vi "franch_sliding_correlator.vi"(4 "error in (no error)":errorcluster, 5 "modulation parameters":T1={"modulation type"="QPSK", "pulse shaping parameters"={"modulation type"=enum."PSK", "pulse shaping filter"=enum."Root Raised Cos", "filter parameter"=0.5, "filter length (symbols)"=8}, "control information\nfor packet header/tail"={"Training Sequence (derived)"=[0.7071067811865475+0.7071067811865475i, 0.7071067811865475+0.7071067811865475i, 0.7071067811865475+0.7071067811865475i, -0.7071067811865475-0.7071067811865475i, -0.7071067811865475-0.7071067811865475i, -0.7071067811865475-0.7071067811865475i, 0.7071067811865475+0.7071067811865475i, -0.7071067811865475-0.7071067811865475i, -0.7071067811865475-0.7071067811865475i, 0.7071067811865475+0.7071067811865475i, -0.7071067811865475-0.7071067811865475i, 0.7071067811865475+0.7071067811865475i, 0.7071067811865475+0.7071067811865475i, 0.7071067811865475+0.7071067811865475i, -0.7071067811865475-0.7071067811865475i, -0.7071067811865475-0.7071067811865475i, -0.7071067811865475-0.7071067811865475i, 0.7071067811865475+0.7071067811865475i, -0.7071067811865475-0.7071067811865475i, -0.7071067811865475-0.7071067811865475i, 0.7071067811865475+0.7071067811865475i, -0.7071067811865475-0.7071067811865475i, 0.7071067811865475+0.7071067811865475i, 0.7071067811865475+0.7071067811865475i, 0.7071067811865475+0.7071067811865475i, -0.7071067811865475-0.7071067811865475i, -0.7071067811865475-0.7071067811865475i, -0.7071067811865475-0.7071067811865475i, 0.7071067811865475+0.7071067811865475i, -0.7071067811865475-0.7071067811865475i, -0.7071067811865475-0.7071067811865475i, 0.7071067811865475+0.7071067811865475i, -0.7071067811865475-0.7071067811865475i, 0.7071067811865475+0.7071067811865475i, 0.7071067811865475+0.7071067811865475i, 0.7071067811865475+0.7071067811865475i, -0.7071067811865475-0.7071067811865475i, -0.7071067811865475-0.7071067811865475i, -0.7071067811865475-0.7071067811865475i, 0.7071067811865475+0.7071067811865475i, -0.7071067811865475-0.7071067811865475i, -0.7071067811865475-0.7071067811865475i, 0.7071067811865475+0.7071067811865475i, -0.7071067811865475-0.7071067811865475i], "Zero Pad Length"=8}, "RX oversample factor"=20, "channel estimation/equalizer\nparameters"={"channel estimate length"=1, "equalizer length"=1, "equalizer delay"=-1, "Equalization Method"="Direct"}, "synchronization options"={"Symbol Timing Recovery Method"="Max Energy", "Synchronization Method"="Timing Estimation", "Correct Frequency Offset"=FALSE, "fixed offset"=0, "Frame Detection Method"="Sliding Correlator"}, "number of data \nsymbols (derived)"=100, "RX Sample Rate"=4000000.0} {"RX Sample Rate" items=["25M"=25000000.0, "20M"=20000000.0, "16.6667M"=16666666.666667, "14.2857M"=14285714.285714, "12.5M"=12500000.0, "11.1111M"=11111111.111111, "10M"=10000000.0, "9.09091M"=9090909.090909, "8.33333M"=8333333.333333, "7.69231M"=7692307.692308, "7.14286M"=7142857.142857, "6.66667M"=6666666.666667, "6.25M"=6250000.0, "5.88235M"=5882352.941176, "5.55556M"=5555555.555556, "5.26316M"=5263157.894737, "5M"=5000000.0, "4.7619M"=4761904.761905, "4.54545M"=4545454.545455, "4.34783M"=4347826.086957, "4.16667M"=4166666.666667, "4M"=4000000.0, "3.84615M"=3846153.846154, "3.7037M"=3703703.703704, "3.57143M"=3571428.571429, "3.44828M"=3448275.862069, "3.33333M"=3333333.333333, "3.22581M"=3225806.451613, "3.125M"=3125000.0, "3.0303M"=3030303.030303, "2.94118M"=2941176.470588, "2.85714M"=2857142.857143, "2.77778M"=2777777.777778, "2.7027M"=2702702.702703, "2.63158M"=2631578.947368, "2.5641M"=2564102.564103, "2.5M"=2500000.0, "2.43902M"=2439024.390244, "2.38095M"=2380952.380952, "2.32558M"=2325581.395349, "2.27273M"=2272727.272727, "2.22222M"=2222222.222222, "2.17391M"=2173913.043478, "2.12766M"=2127659.574468, "2.08333M"=2083333.333333, "2.04082M"=2040816.326531, "2M"=2000000.0, "1.96078M"=1960784.313725, "1.92308M"=1923076.923077, "1.88679M"=1886792.45283, "1.85185M"=1851851.851852, "1.81818M"=1818181.818182, "1.78571M"=1785714.285714, "1.75439M"=1754385.964912, "1.72414M"=1724137.931034, "1.69492M"=1694915.254237, "1.66667M"=1666666.666667, "1.63934M"=1639344.262295, "1.6129M"=1612903.225806, "1.5873M"=1587301.587302, "1.5625M"=1562500.0, "1.53846M"=1538461.538462, "1.51515M"=1515151.515152, "1.49254M"=1492537.313433, "1.47059M"=1470588.235294, "1.44928M"=1449275.362319, "1.42857M"=1428571.428571, "1.40845M"=1408450.704225, "1.38889M"=1388888.888889, "1.36986M"=1369863.013699, "1.35135M"=1351351.351351, "1.33333M"=1333333.333333, "1.31579M"=1315789.473684, "1.2987M"=1298701.298701, "1.28205M"=1282051.282051, "1.26582M"=1265822.78481, "1.25M"=1250000.0, "1.23457M"=1234567.901235, "1.21951M"=1219512.195122, "1.20482M"=1204819.277108, "1.19048M"=1190476.190476, "1.17647M"=1176470.588235, "1.16279M"=1162790.697674, "1.14943M"=1149425.287356, "1.13636M"=1136363.636364, "1.1236M"=1123595.505618, "1.11111M"=1111111.111111, "1.0989M"=1098901.098901, "1.08696M"=1086956.521739, "1.07527M"=1075268.817204, "1.06383M"=1063829.787234, "1.05263M"=1052631.578947, "1.04167M"=1041666.666667, "1.03093M"=1030927.835052, "1.02041M"=1020408.163265, "1.0101M"=1010101.010101, "1M"=1000000.0, "990.099k"=990099.009901, "980.392k"=980392.156863, "970.874k"=970873.786408, "961.538k"=961538.461538, "952.381k"=952380.952381, "943.396k"=943396.226415, "934.579k"=934579.439252, "925.926k"=925925.925926, "917.431k"=917431.192661, "909.091k"=909090.909091, "900.901k"=900900.900901, "892.857k"=892857.142857, "884.956k"=884955.752212, "877.193k"=877192.982456, "869.565k"=869565.217391, "862.069k"=862068.965517, "854.701k"=854700.854701, "847.458k"=847457.627119, "840.336k"=840336.134454, "833.333k"=833333.333333, "826.446k"=826446.280992, "819.672k"=819672.131148, "813.008k"=813008.130081, "806.452k"=806451.612903, "800k"=800000.0, "793.651k"=793650.793651, "787.402k"=787401.574803, "781.25k"=781250.0, "769.231k"=769230.769231, "757.576k"=757575.757576, "746.269k"=746268.656716, "735.294k"=735294.117647, "724.638k"=724637.681159, "714.286k"=714285.714286, "704.225k"=704225.352113, "694.444k"=694444.444444, "684.932k"=684931.506849, "675.676k"=675675.675676, "666.667k"=666666.666667, "657.895k"=657894.736842, "649.351k"=649350.649351, "641.026k"=641025.641026, "632.911k"=632911.392405, "625k"=625000.0, "617.284k"=617283.950617, "609.756k"=609756.097561, "602.41k"=602409.638554, "595.238k"=595238.095238, "588.235k"=588235.294118, "581.395k"=581395.348837, "574.713k"=574712.643678, "568.182k"=568181.818182, "561.798k"=561797.752809, "555.556k"=555555.555556, "549.451k"=549450.549451, "543.478k"=543478.26087, "537.634k"=537634.408602, "531.915k"=531914.893617, "526.316k"=526315.789474, "520.833k"=520833.333333, "515.464k"=515463.917526, "510.204k"=510204.081633, "505.051k"=505050.505051, "500k"=500000.0, "495.05k"=495049.50495, "490.196k"=490196.078431, "485.437k"=485436.893204, "480.769k"=480769.230769, "476.19k"=476190.47619, "471.698k"=471698.113208, "467.29k"=467289.719626, "462.963k"=462962.962963, "458.716k"=458715.59633, "454.545k"=454545.454545, "450.45k"=450450.45045, "446.429k"=446428.571429, "442.478k"=442477.876106, "438.596k"=438596.491228, "434.783k"=434782.608696, "431.034k"=431034.482759, "427.35k"=427350.42735, "423.729k"=423728.813559, "420.168k"=420168.067227, "416.667k"=416666.666667, "413.223k"=413223.140496, "409.836k"=409836.065574, "406.504k"=406504.065041, "403.226k"=403225.806452, "400k"=400000.0, "396.825k"=396825.396825, "393.701k"=393700.787402, "390.625k"=390625.0, "384.615k"=384615.384615, "378.788k"=378787.878788, "373.134k"=373134.328358, "367.647k"=367647.058824, "362.319k"=362318.84058, "357.143k"=357142.857143, "352.113k"=352112.676056, "347.222k"=347222.222222, "342.466k"=342465.753425, "337.838k"=337837.837838, "333.333k"=333333.333333, "328.947k"=328947.368421, "324.675k"=324675.324675, "320.513k"=320512.820513, "316.456k"=316455.696203, "312.5k"=312500.0, "308.642k"=308641.975309, "304.878k"=304878.04878, "301.205k"=301204.819277, "297.619k"=297619.047619, "294.118k"=294117.647059, "290.698k"=290697.674419, "287.356k"=287356.321839, "284.091k"=284090.909091, "280.899k"=280898.876404, "277.778k"=277777.777778, "274.725k"=274725.274725, "271.739k"=271739.130435, "268.817k"=268817.204301, "265.957k"=265957.446809, "263.158k"=263157.894737, "260.417k"=260416.666667, "257.732k"=257731.958763, "255.102k"=255102.040816, "252.525k"=252525.252525, "250k"=250000.0, "247.525k"=247524.752475, "245.098k"=245098.039216, "242.718k"=242718.446602, "240.385k"=240384.615385, "238.095k"=238095.238095, "235.849k"=235849.056604, "233.645k"=233644.859813, "231.481k"=231481.481481, "229.358k"=229357.798165, "227.273k"=227272.727273, "225.225k"=225225.225225, "223.214k"=223214.285714, "221.239k"=221238.938053, "219.298k"=219298.245614, "217.391k"=217391.304348, "215.517k"=215517.241379, "213.675k"=213675.213675, "211.864k"=211864.40678, "210.084k"=210084.033613, "208.333k"=208333.333333, "206.612k"=206611.570248, "204.918k"=204918.032787, "203.252k"=203252.03252, "201.613k"=201612.903226, "200k"=200000.0, "198.413k"=198412.698413, "196.85k"=196850.393701, "195.312k"=195312.5]; "control information\nfor packet header/tail"."Training Sequence (derived)" format="%#_3p"}, 7 "input complex waveform":cluster{"t0":dbl, "dt":dbl, "Y":cdb[]}={"t0"=0.0, "dt"=1.0, "Y"=[]} {"Y" format="%.3f"; "dt" format="%^.2e"; "t0" format="%.4f"}) -> (0 "error out":errorcluster, 1 "frequency offset":dbl format="%#_6p", 2 "frame offset":i32, 3 "output":cdb[](array[numeric]) format="%#_3p")   [LabVIEW 2012]
uses:
  lab5/control_type_defs.llb/rx_modulation params.ctl
  <vilib>/Analysis/2dsp.llb/1D Cross Correlation (CDB).vi
  <vilib>/Analysis/NI_AALPro.lvlib
  <vilib>/Analysis/NI_AAL_SigProc.lvlib
panel:
  out "Correlation":cdb[](array[numeric])
  out "subarray":cdb[](array[numeric])
  out "x^2":dbl[](array[numeric])
  out "max index(es)":i32
  out "x/y":dbl
  out "output array":cdb[](array[numeric])
  out "x-y":dbl
  # "( set delay to -1 for equalizer\n  to choose optimal delay )"
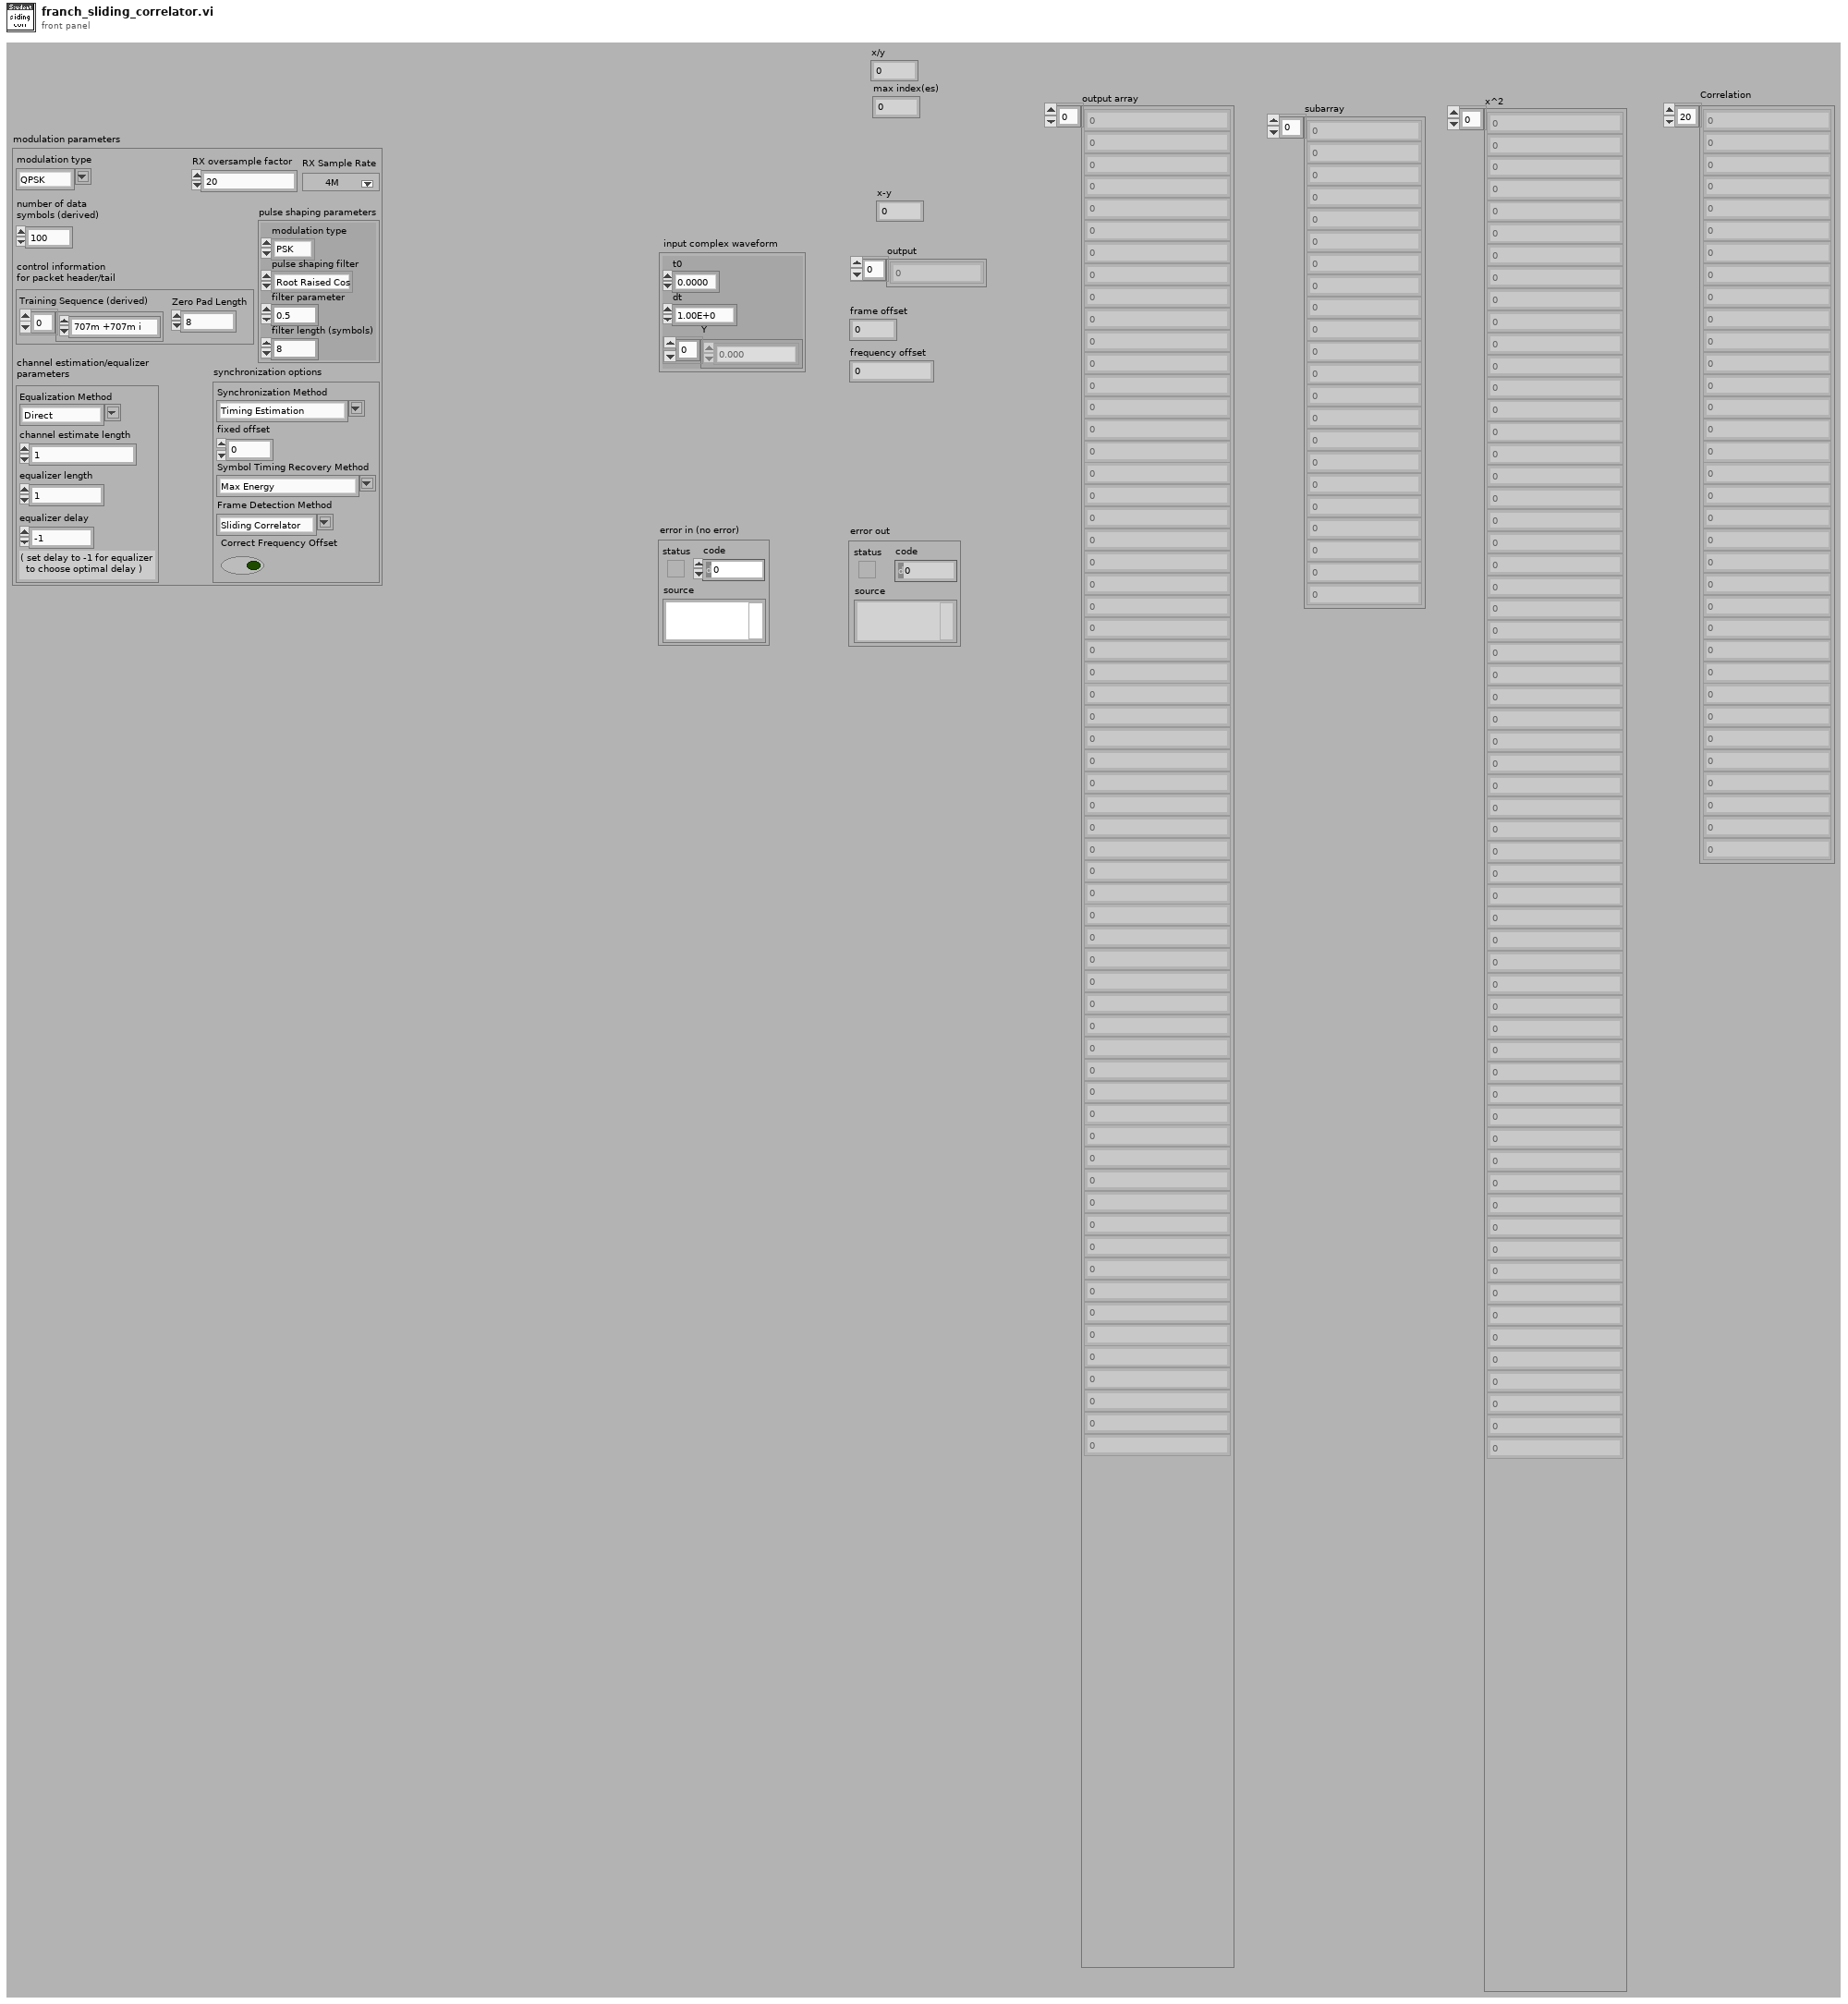
[diagram p1: front panel]
types:
  T1 = typedef "rx_modulation params.ctl" = cluster{"modulation type":string, "pulse shaping parameters":cluster{"modulation type":enum16{"FSK", "PSK", "QAM", "MSK", "PAM", "ASK"}, "pulse shaping filter":enum16{"none", "Raised Cosine", "Root Raised Cos", "Gaussian"}, "filter parameter":dbl, "filter length (symbols)":i32}, "control information\nfor packet header/tail":cluster{"Training Sequence (derived)":cdb[], "Zero Pad Length":i32}, "RX oversample factor":i32, "channel estimation/equalizer\nparameters":cluster{"channel estimate length":i32, "equalizer length":i32, "equalizer delay":i32, "Equalization Method":string}, "synchronization options":cluster{"Symbol Timing Recovery Method":string, "Synchronization Method":string, "Correct Frequency Offset":bool, "fixed offset":i32, "Frame Detection Method":string}, "number of data \nsymbols (derived)":i32, "RX Sample Rate":dbl}
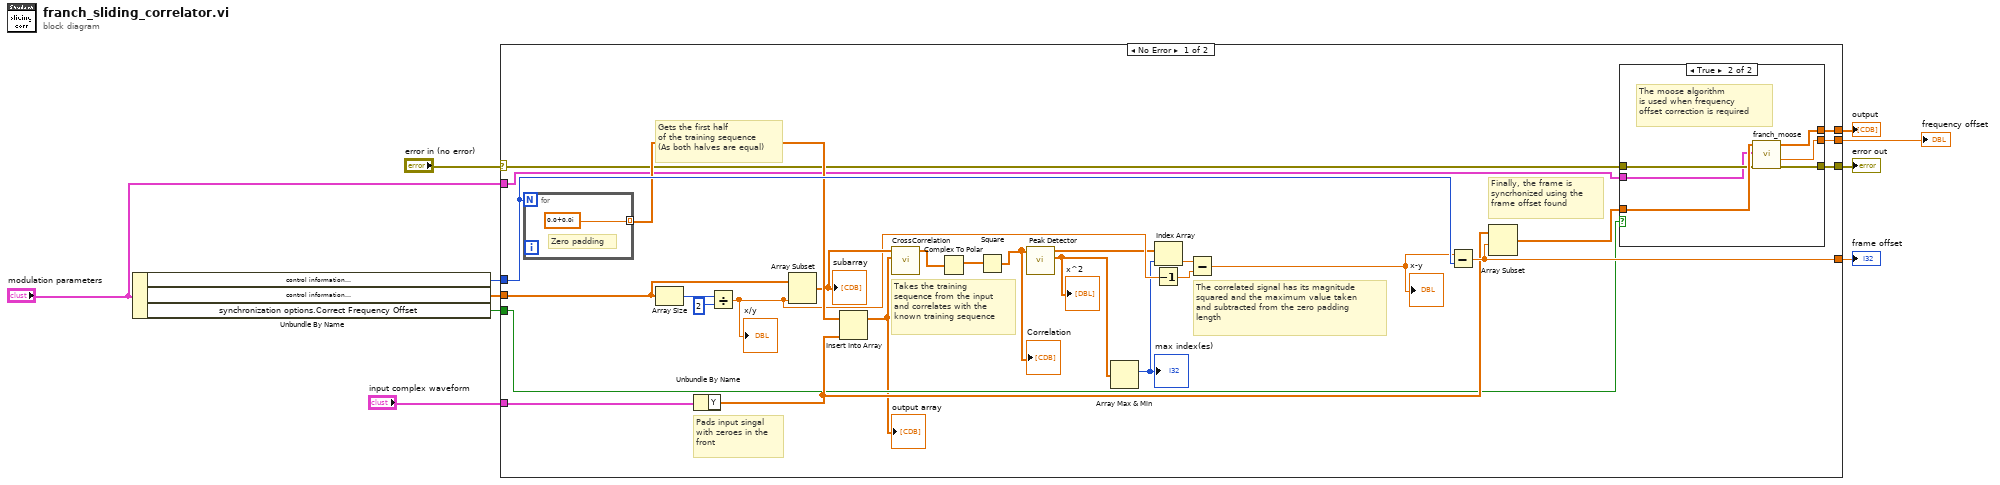
[diagram p0: block diagram]
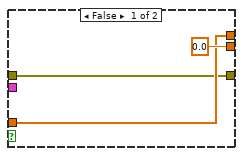
[diagram p2: hidden frame]
diagram:
  n1 = Unbundle By Name("modulation parameters") -> ("control information\nfor packet header/tail.Zero Pad Length"=w1:i32, "control information\nfor packet header/tail.Training Sequence (derived)"=w5:cdb[], "synchronization options.Correct Frequency Offset"=w8:bool)
  n2 = case shown="No Error" "error in (no error)" {
    selector: "error in (no error)" -> [w29 w48]
    tunnel: [w28 w48] -> w9
    tunnel: w8 -> [w32 _]
    tunnel: "modulation parameters" -> [w27 _]
    tunnel: "input complex waveform" -> [w37 _]
    tunnel: w5 -> [w11 _]
    tunnel: [w26 _] -> w4
    tunnel: [w30 _] -> w3
    tunnel: [w35 _] -> w2
    tunnel: w1 -> [w36 _]
    frame No Error {
      # "Finally, the frame is\nsyncrhonized using the\nframe offset found"
      # "Takes the training\nsequence from the input\nand correlates with the\nknown training sequence"
      # "The correlated signal has its magnitude\nsquared and the maximum value taken \nand subtracted from the zero padding \nlength"
      # "Pads input singal\nwith zeroes in the \nfront"
      # "Gets the first half\nof the training sequence\n(As both halves are equal)"
      n3 = for {
        N: w36 -> [_]
        tunnel: [cdb 0.0+0.0i] -> w34 mode=indexing
        # "Zero padding"
      }
      n4 = Array Size(array=w11) -> (size(s)=w25:i32)
      n5 = Unbundle By Name(w37) -> ("Y"=w33:cdb[])
      n6 = Divide(x=w25, y=2) -> (x/y=w20:dbl)
      "x/y" <- w20
      n7 = Array Subset(array=w11, length=w20) -> (w24:cdb[])  [unwired: 1 in]
      "subarray" <- w24
      n8 = Insert Into Array(array=w34, new element=w33) -> (w23:cdb[])  [unwired: 1 in]
      "output array" <- w23
      n9 = call-poly <vilib>:"CrossCorrelation.vi"("Y"=w23, "X"=w24) -> ("Rxy"=w14:cdb[])  [unwired: 8 in, 1 out]
      n10 = Complex To Polar(r * e^(i*theta)=w14) -> (r=w13:dbl[])  [unwired: 1 out]
      n11 = Square(x=w13) -> (x^2=w12:dbl[])
      "Correlation" <- w12
      n12 = call <vilib>:"Peak Detector.vi"("X"=w12) -> ("Amplitudes"=w22:dbl[], "Locations"=w16:dbl[])  [unwired: 6 in, 3 out]
      "x^2" <- w22
      n13 = Array Max & Min(array=w22) -> (max index (indices)=w17:i32)  [unwired: 3 out]
      "max index(es)" <- w17
      n14 = Decrement(x=w20) -> (x-1=w18:dbl)
      n15 = Index Array(array=w16, index=w17) -> (element=w15:dbl)
      n16 = Subtract(x=w15, y=w18) -> (x-y=w19:dbl)
      "x-y" <- w19
      n17 = Subtract(x=w19, y=w36) -> (x-y=w35:dbl)
      n18 = Array Subset(array=w33, index=w35) -> (w31:cdb[])  [unwired: 1 in]
      n19 = case shown="True" w32 {
        tunnel: w31 -> [w39 w46]
        tunnel: [w39 w45] -> w30
        tunnel: w29 -> [w38 w44]
        tunnel: [w38 w43] -> w28
        tunnel: w27 -> [_ w42]
        tunnel: [0.0 ("frequency offset") w41] -> w26
        frame False {
        }
        frame True {
          # "The moose algorithm\nis used when frequency\noffset correction is required"
          n20 = call "franch_moose.vi"("error in (no error)"=w44, "modulation parameters"=w42, "input"=w46) -> ("error out"=w43:errorcluster, "frequency offset"=w41:dbl, "output"=w45:cdb[])  [unwired: 2 in]
        }
      }
    }
    frame Error {
    }
  }
  "error out" <- w9
  "output" <- w3
  "frequency offset" <- w4
  "frame offset" <- w2
